vi "Database Logging.vi"() -> ()   [LabVIEW 2023]
doc: "This example inserts data into a table named logging in the LabVIEW.mdb database. The data is generated and inserted into the database once per second until you press the Stop button. You can use either of the Playback examples to read the data back into LabVIEW.\n\nThe diagram is easy to use because you only need three Database Tools subVIs - DB Tools Open Connection, DB Tools Insert Data, and DB Tools Close Connection. To insert the data, you do not need to use SQL commands or worry about defining or converting data types. You bundle all the data into a cluster and wire that cluster to the DB Tools Insert Data VI."
uses:
  <vilib>/addons/database/Connection.llb/DB Tools Open Connec (Path).vi
  <vilib>/addons/database/NI_Database_API.lvlib
panel:
  out "Number of Records":i32
  in  "Stop":bool
  out "min temperature value":dbl format="%#.6g"
  out "max temperature value":dbl format="%#.6g"
  out "min pressure value":dbl format="%#.6g"
  out "max pressure value":dbl format="%#.6g"
  out "Core Temperature":dbl[](graph)
  out "Core Pressure":dbl[](graph)
  # "Overview: Demonstrates the use of the DB Tools Insert Data VI to insert data into a database.\nRequirements: Database Connectivity Toolkit\nInstructions:\n1. Run the VI to log data to the example database.\n2. Open one of the \"Playback\" database examples to display the data that was logged."
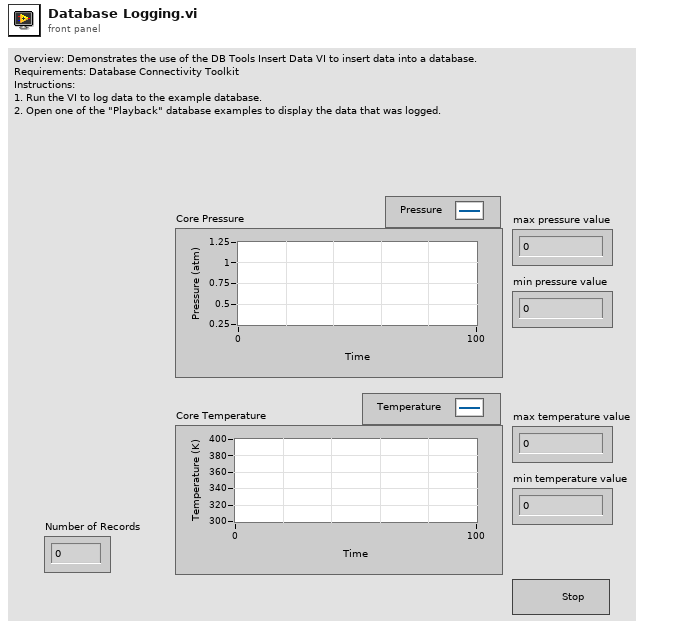
[diagram p1: front panel]
types:
  T1 = typedef "NI_Database_API.lvlib/Conn ObjectReference.ctl" = refnum<k1>
  T2 = cluster{i32, "core pressure":dbl[], dbl, dbl, "core temperature":dbl[], dbl, dbl}
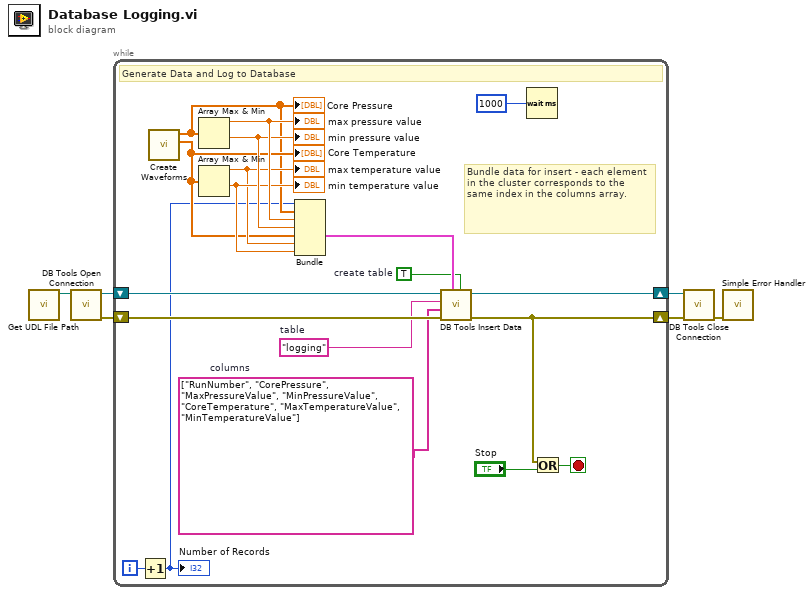
[diagram p0: block diagram]
diagram:
  n1 = call "Get UDL File Path.vi"() -> ("UDL file path"=w1:path)  [unwired: 11 in]
  n2 = call-poly <vilib>:"DB Tools Open Connection.vi"("connection information"=w1) -> ("error out"=w5:errorcluster, "connection reference"=w6:T1)  [unwired: 7 in]
  n3 = while {
    shift-right: [w9] -> w3
    shift-left: w5 -> [w18]
    shift-right: [w20] -> w4
    shift-left: w6 -> [w19]
    i -> [w21]
    stop <- w14 stop-if-true
    w7 = string[] ["RunNumber", "CorePressure", "MaxPressureValue", "MinPressureValue", "CoreTemperature", "MaxTemperatureValue", "MinTemperatureValue"]  # columns
    w8 = "logging"  # table
    w16 = TRUE  # create table
    # "Bundle data for insert - each element in the cluster corresponds to the same index in the columns array."
    # "Generate Data and Log to Database"
    n4 = Increment(x=w21) -> (x+1=w11:i32)
    "Number of Records" <- w11
    n5 = call "Create Waveforms.vi"() -> ("core temperature"=w13:dbl[], "core pressure"=w12:dbl[])  [unwired: 10 in]
    "Core Pressure" <- w12
    "Core Temperature" <- w13
    n6 = Array Max & Min(array=w12) -> (max value=w25:dbl, min value=w24:dbl)  [unwired: 2 out]
    "max pressure value" <- w25
    "min pressure value" <- w24
    n7 = Array Max & Min(array=w13) -> (max value=w22:dbl, min value=w23:dbl)  [unwired: 2 out]
    "max temperature value" <- w22
    "min temperature value" <- w23
    n8 = Bundle(w11, "core pressure"=w12, w25, w24, "core temperature"=w13, w22, w23) -> (w17:T2)  [unwired: 1 in]
    n9 = call <vilib>:"DB Tools Insert Data.vi"("create table? (F)"=w16, "data"=w17, "error in (no error)"=w18, "columns"=w7, "table"=w8, "connection reference"=w19) -> ("error out"=w9:errorcluster, "connection reference out"=w20:T1)  [unwired: 4 in]
    n10 = Wait (ms)(milliseconds to wait=u32 1000) -> ()  [unwired: 1 out]
    n11 = Or(x=w9, y="Stop") -> (x .or. y?=w14:bool)
  }
  n12 = call <vilib>:"DB Tools Close Connection.vi"("error in (no error)"=w3, "connection reference"=w4) -> ("error out"=w2:errorcluster)  [unwired: 5 in]
  n13 = call <vilib>:"Simple Error Handler.vi"("error in (no error)"=w2) -> ()  [unwired: 4 in, 5 out]
